vi "Definition Cluster.vi"(11 "Relation in":refnum<class "Relation.lvclass">) -> (2 "Definition":variant, 3 "Relation out":refnum<class "Relation.lvclass">)   [LabVIEW 2020, in "Conditum.lvlib" / "Columns.lvlib" / "Relation.lvclass"]
uses:
  Relation.lvclass
  C:/dev/lv20CE/lv-conditum/Conditum/Columns/Type/Type.lvclass
  Relation Definition.ctl
  Type/Definition.ctl
  Relation Info.ctl
  Relation Mapping.ctl
  Conditum.lvlib
  Type/Type.lvclass
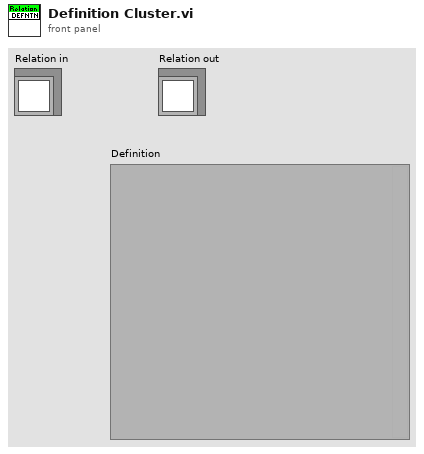
[diagram p1: front panel]
types:
  T1 = typedef "Conditum.lvlib/Columns.lvlib/Relation.lvclass/Relation Definition.ctl" = cluster{"Type":T2, "Relation":T3}
  T2 = typedef "Conditum.lvlib/Columns.lvlib/Type.lvclass/Definition.ctl" = cluster{"Name":string, "Nullable":bool, "Default NULL":bool}
  T3 = typedef "Conditum.lvlib/Relation Info.ctl" = cluster{"Mapping":T4, "Related To":string, "Reversed By":string}
  T4 = typedef "Conditum.lvlib/Relation Mapping.ctl" = enum16{"OneToOne", "OneToMany", "ManyToOne", "ManyToMany"}
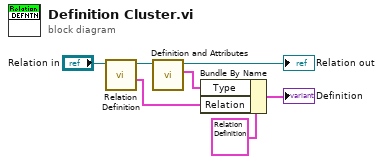
[diagram p0: block diagram]
diagram:
  n1 = call "Relation Definition.vi"("Relation in"="Relation in") -> ("Relation Definition"=w6:T3, "Relation out"=w4:refnum<class "Relation.lvclass">)  [unwired: 8 in, 1 out]
  n2 = call "Definition and Attributes.vi"("Type in"=w4) -> ("Definition"=w5:T2, "Type out"=→"Relation out":refnum<class "Relation.lvclass">)  [unwired: 8 in, 1 out]
  n3 = Bundle By Name(cluster=T1 {"Type"={"Name"="", "Nullable"=FALSE, "Default NULL"=FALSE}, "Relation"={"Mapping"=enum."OneToMany", "Related To"="", "Reversed By"=""}} ("Relation Definition"), "Type"=w5, "Relation"=w6) -> (→"Definition":T1)
